vi "grSim Packet Command UDP Test.vi"(0 "Robots":T1[](array[typedef]), 9 "SSL Vision Address:":string="127.0.0.1", 11 "Port:":u16=20011) -> (6 "connection ID out":refnum<k16>)   [LabVIEW 2020]
uses:
  Convert AI Robot to Robot Command Folder/grSim/grSim Robot Command.ctl
  Communication.lvclass
panel:
  out "Array":u8[](array[numeric])
  out "error out":errorcluster
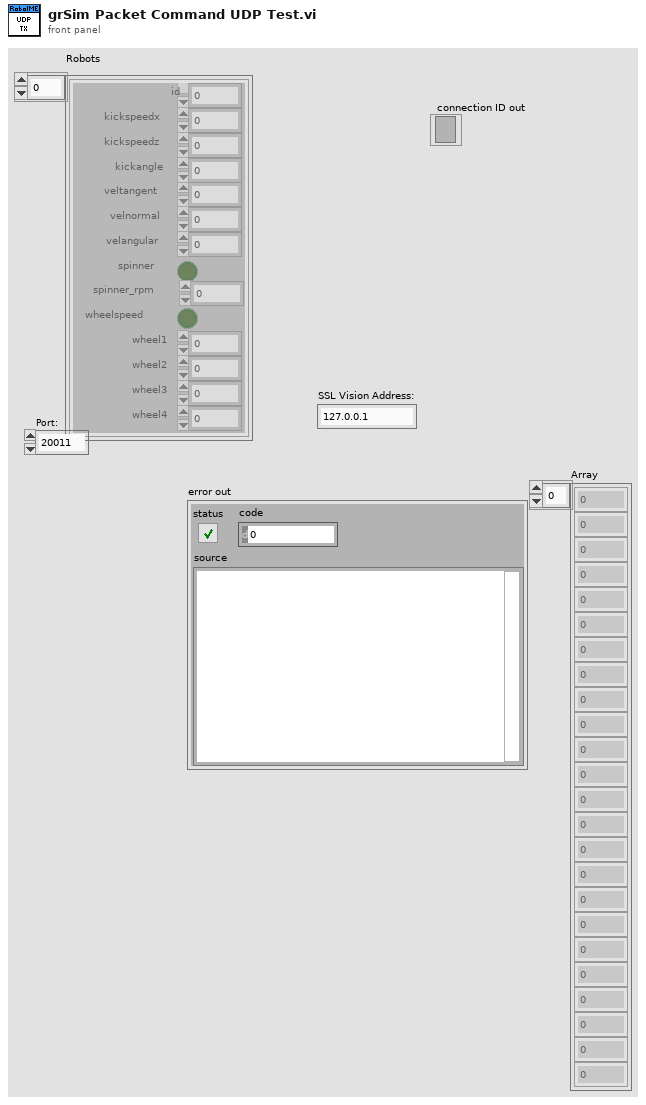
[diagram p1: front panel]
types:
  T1 = typedef "grSim Robot Command.ctl" = cluster{"id":u32, "kickspeedx":sgl, "kickspeedz":sgl, "veltangent":sgl, "velnormal":sgl, "velangular":sgl, "spinner":bool, "wheelspeed":bool, "wheel1":sgl, "wheel2":sgl, "wheel3":sgl, "wheel4":sgl, "kickangle":sgl, "spinner_rpm":sgl}
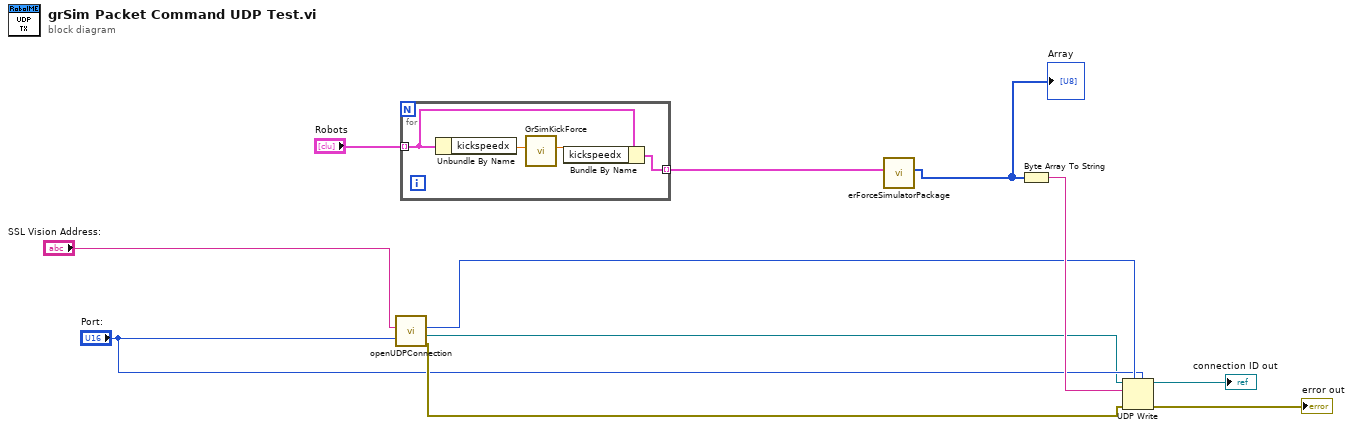
[diagram p0: block diagram]
diagram:
  n1 = call "openUDPConnection.vi"("Port:"="Port:", "SSL Vision Address:"="SSL Vision Address:") -> ("error out"=w4:errorcluster, "connectionID out"=w1:refnum<k16>, "IP Address"=w5:u32)  [unwired: 6 in, 1 out]
  n2 = for {
    tunnel: "Robots" -> [w15] mode=indexing
    tunnel: [w14] -> w9 mode=indexing
    n3 = Unbundle By Name(w15) -> ("kickspeedx"=w13:sgl)
    n4 = call "GrSimKickForce.vi"("real kick"=w13) -> ("grsim kick"=w12:dbl)  [unwired: 10 in]
    n5 = Bundle By Name(cluster=w15, "kickspeedx"=w12) -> (w14:T1)
  }
  n6 = call "erForceSimulatorPackage.vi"("robots"=w9) -> ("robotControl"=w8:u8[])  [unwired: 8 in, 2 out]
  "Array" <- w8
  n7 = Byte Array To String(unsigned byte array=w8) -> (string=w6:string)
  n8 = UDP Write(address=w5, port or service name="Port:", connection ID=w1, data in=w6, 8:w4) -> (error out=→"error out":errorcluster, 3:→"connection ID out":refnum<k16>)  [unwired: 1 in]
